vi "New SSE Client.vi"(7 "Last Event ID (None)":string, 8 "error in (no error)":errorcluster, 10 "SSE Client":refnum<class "SSE Client.lvclass">, 11 "SSE Manager in":refnum<class "SSE Manager.lvclass">) -> (0 "error out":errorcluster, 3 "SSE Manager out":refnum<class "SSE Manager.lvclass">)   [LabVIEW 2020, in "Server Sent Events Example.lvlib" / "SSE Manager.lvclass"]
uses:
  SSE Manager.lvclass
  lv-http-server/HTTP Server/SSE Client/SSE Client.lvclass
  SSE Manager.lvclass/SSE Manager.ctl
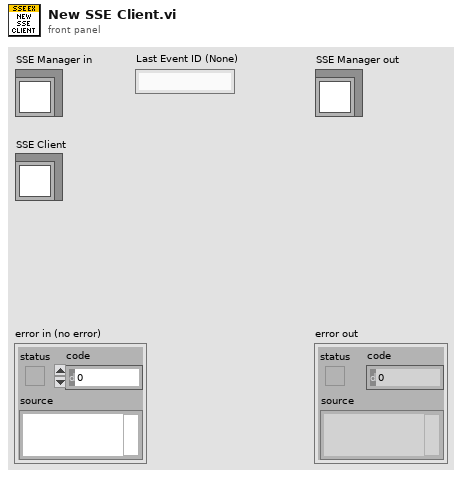
[diagram p1: front panel]
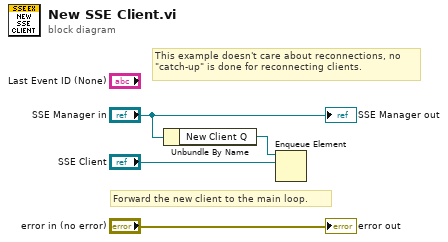
[diagram p0: block diagram]
diagram:
  # "Forward the new client to the main loop."
  # "This example doesn't care about reconnections, no \"catch-up\" is done for reconnecting clients."
  n1 = Unbundle By Name("SSE Manager in") -> ("New Client Q"=w2:refnum<queue>)
  n2 = Enqueue Element(queue=w2, element="SSE Client") -> ()  [unwired: 2 in, 3 out]
  "error out" <- "error in (no error)"
  "SSE Manager out" <- "SSE Manager in"
